vi "_ROSMasterConsole.vi"() -> ()   [LabVIEW 2012]
uses:
  <vilib>/Utility/miscctls.llb/LVRectTypeDef.ctl
  <userlib>/ROSforLV/ROS/Code/_ROSDefinition.vi
  <vilib>/Utility/cursorutil.llb/Set Cursor (Icon Pict).vi
panel:
  out "Servers Closed":bool[](array[boolean])
  in  "Stop":bool
  out "Error Log":string
  out "ROS Master":string="192.168.1.110:11311"
  out "selection":i32=-1
  out "2D Picture":picture
  out "Boundaries":cluster{i32, i32}[](array[cluster])=[{10, 22}, {30, 42}, {50, 62}]
  in  "expand?":bool
  out "Status":string
  out "Master?":bool
  out "Running?":bool
  out "current task":string
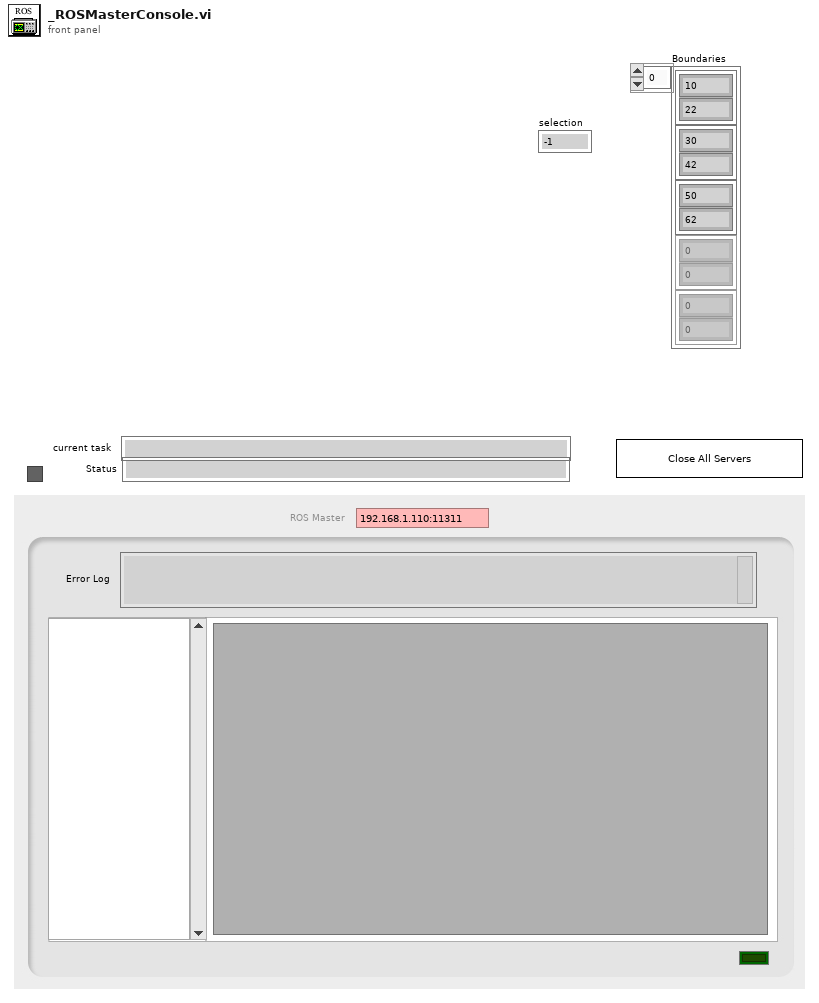
[diagram p1: front panel]
types:
  T1 = enum16{"Add Server", "Clear Server", "Clear All", "Get Info"}
  T2 = enum16{"Get Nodes", "Start Nodes", "Reset Nodes"}
  T3 = typedef "LVRectTypeDef.ctl" = cluster{"Left":i16, "Top":i16, "Right":i16, "Bottom":i16}
  T4 = typedef "_ROSControl.ctl" = cluster{"topic port":u16, "Node":string, "topic":string, "type":string, "node port":u32, "error ":errorcluster, "Direction":T5, "APIs":string[], "Update (ms)":u16, "write queue":u16}
  T5 = typedef "_ROSDirection.ctl" = enum16{"Node", "Publisher", "Subscriber", "Service Client"}
  T6 = typedef "ServoInfo.ctl" = cluster{"vi name":string, "VI Refnum":refnum<vi>, "queue":refnum<queue>, "ROS":T4, "notifier":refnum<notifier>}
  T7 = typedef "LVMouseTypeDef.ctl" = cluster{"Mouse Position":cluster{"X":i32, "Y":i32}, "Mouse Modifiers":cluster{"Button Down":bool, "Shift Mod":bool, "Menu Mod":bool, "Option Mod":bool}}
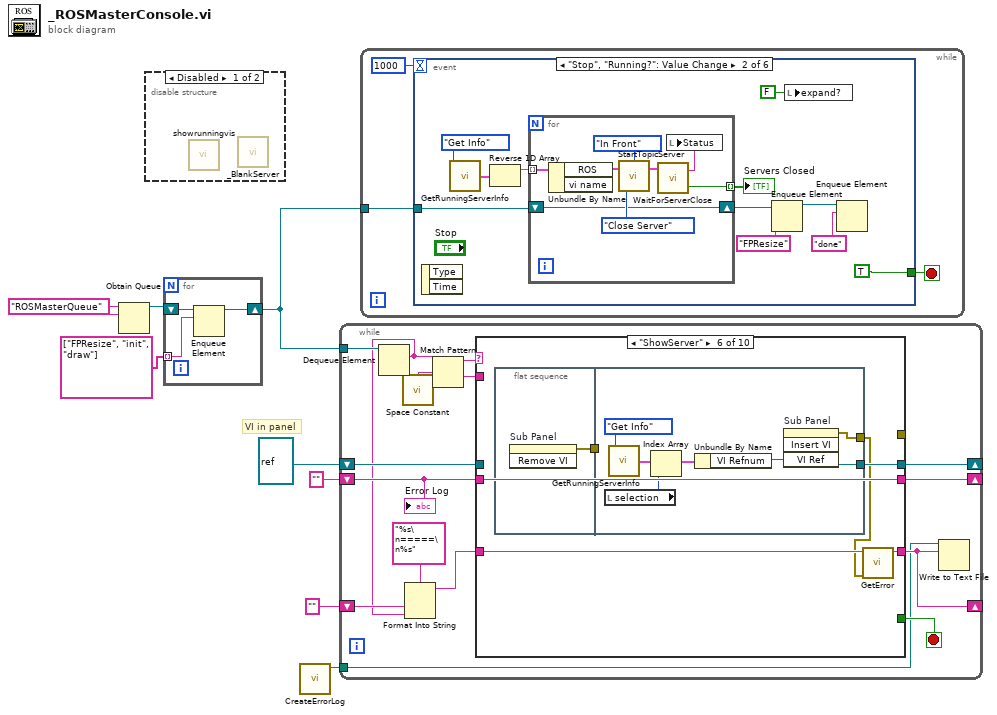
[diagram p0: block diagram]
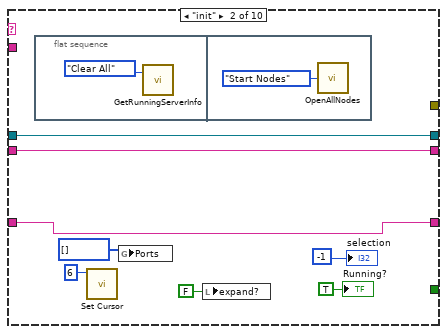
[diagram p4: hidden frame]
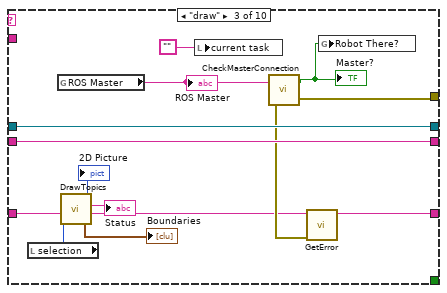
[diagram p5: hidden frame]
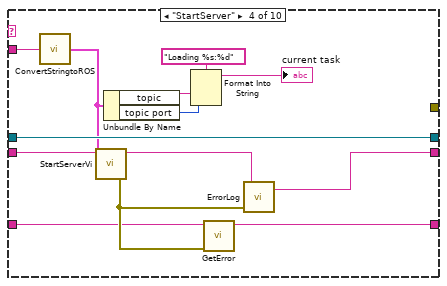
[diagram p6: hidden frame]
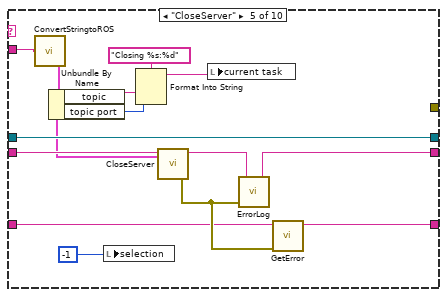
[diagram p7: hidden frame]
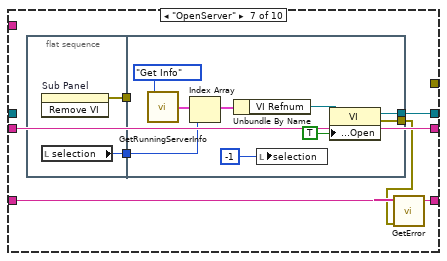
[diagram p8: hidden frame]
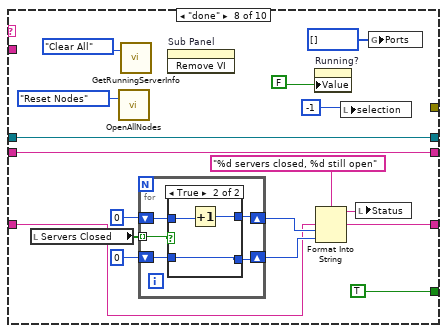
[diagram p9: hidden frame]
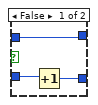
[diagram p10: hidden frame]
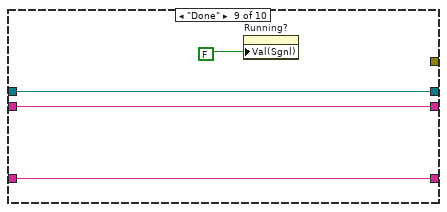
[diagram p11: hidden frame]
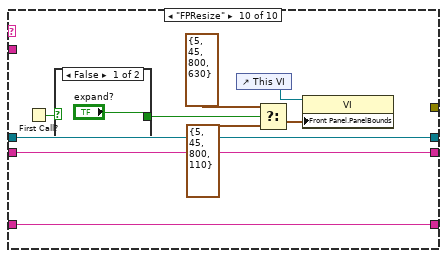
[diagram p12: hidden frame]
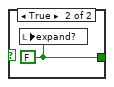
[diagram p13: hidden frame]
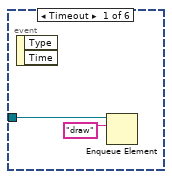
[diagram p14: hidden frame]
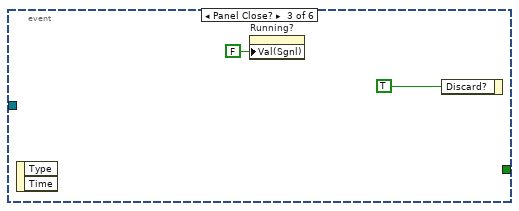
[diagram p15: hidden frame]
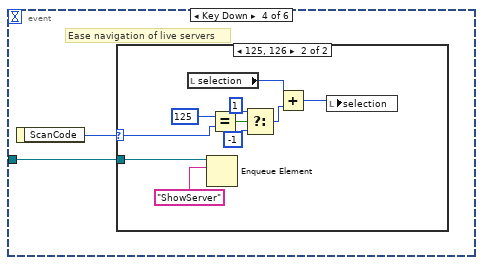
[diagram p16: hidden frame]
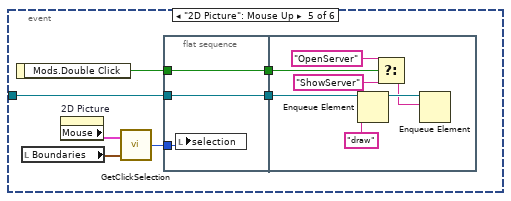
[diagram p18: hidden frame]
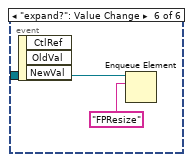
[diagram p19: hidden frame]
diagram:
  w8 = "ROSMasterQueue" ("name (unnamed)")
  # "VI in panel"
  n1 = Obtain Queue(name (unnamed)=w8, element data type=w8) -> (queue out=w5:refnum<queue>)  [unwired: 3 in, 2 out]
  n2 = disable-structure shown="Disabled" {
    frame Disabled {
      n3 = call <userlib>:"showrunningvis.vi"() -> ()  [unwired: 1 in]
      n4 = call <userlib>:"_BlankServer.vi"() -> ()  [unwired: 4 in]
    }
    frame Enabled {
    }
  }
  n5 = for {
    shift-right: [w11] -> w7
    shift-left: w5 -> [w10]
    tunnel: string[] ["FPResize", "init", "draw"] -> [w9] mode=indexing
    n6 = Enqueue Element(queue=w10, element=w9) -> (queue out=w11:refnum<queue>)  [unwired: 2 in, 2 out]
  }
  n7 = call <userlib>:"CreateErrorLog.vi"() -> ("path"=w1:path)  [unwired: 11 in]
  n8 = while {
    tunnel: w7 -> [w26]
    shift-right: [w20] -> _
    shift-left: refnum<vi> refnum ("VI Ref") -> [w21]
    shift-right: [w19] -> _
    shift-left: "" ("String out") -> [w18]
    shift-right: [w13] -> _
    shift-left: "" -> [w17]
    tunnel: w1 -> [w12]
    stop <- w25 stop-if-true
    n9 = Dequeue Element(queue=w26) -> (element=w15:string)  [unwired: 2 in, 3 out]
    n10 = call <vilib>:"Space Constant.vi"() -> ("String"=w23:string)
    n11 = Format Into String(format string="%s\n=====\n%s", w17, w15) -> (resulting string=w14:string)  [unwired: 2 in, 1 out]
    n12 = Match Pattern(string=w15, regular expression=w23) -> (before substring=w24:string, after substring=w22:string)  [unwired: 1 in, 2 out]
    n13 = case shown="\"ShowServer\"" w24 {
      tunnel: [_ _ _ _ _ _ _ TRUE _ _] -> w25
      tunnel: w22 -> [_ _ _ w60 w69 _ _ _ _ _]
      tunnel: w21 -> [w29 w37 w51 w63 w76 _ _ w122 w138 w147]
      tunnel: [w29 w37 w51 w63 w76 w81 w94 w122 w138 w147] -> w20
      tunnel: [_ _ w42 _ _ _ _ _ _ _] -> _
      tunnel: [w28 w31 w47 w55 w73 w80 w93 w117 w136 w140] -> w19
      tunnel: w18 -> [w28 w31 w47 w56 w74 w80 w93 w117 w136 w140]
      tunnel: w14 -> [w27 w30 w41 w53 w64 w78 w91 w108 w135 w139]
      tunnel: [w27 w30 w40 w52 w66 w79 w92 w108 w135 w139] -> w13
      frame Default {
      }
      frame "init" {
        n14 = flat-sequence {
          frame #0 {
            n15 = call <userlib>:"GetRunningServerInfo.vi"("Task"=T1."Clear All") -> ()  [unwired: 1 in, 3 out]
          }
          frame #1 {
            n16 = call <userlib>:"OpenAllNodes.vi"("Task"=T2."Start Nodes") -> ()  [unwired: 1 in, 1 out]
          }
        }
        n17 = call-poly <vilib>:"Set Cursor.vi"("icon"=u16 6) -> ()  [unwired: 9 in, 2 out]
        n18 = global write "_ROSDefinition.vi" "Ports"(u16[] [] ("Ports")) -> ()
        n19 = local write "expand?"(FALSE ("expand?")) -> ()
        "Running?" <- TRUE ("Running?")
        "selection" <- -1 ("selection")
      }
      frame "draw" {
        n20 = local read "selection"() -> (w50:i32)
        n21 = global read "_ROSDefinition.vi" "ROS Master"() -> (w45:string)
        "ROS Master" <- w45
        n22 = call <userlib>:"DrawTopics.vi"("Selection"=w50) -> ("new picture"=→"2D Picture":picture, "Status"=→"Status":string, "Boundaries"=→"Boundaries":cluster{i32, i32}[])  [unwired: 2 in, 1 out]
        n23 = local write "current task"("") -> ()
        n24 = call <userlib>:"CheckMasterConnection.vi"("Master IP"=w45) -> ("error out"=w42:errorcluster, "Master There?"=w43:bool)  [unwired: 1 in]
        "Master?" <- w43
        n25 = call <userlib>:"GetError.vi"("error in (no error)"=w42, "String in"=w41) -> ("String out"=w40:string)  [unwired: 9 in]
        n26 = global write "_ROSDefinition.vi" "Robot There?"(w43) -> ()
      }
      frame "StartServer" {
        n27 = call <userlib>:"ConvertStringtoROS.vi"("string in"=w60) -> ("ROS"=w57:T4)
        n28 = call <userlib>:"StartServerVi.vi"("ROS in"=w57) -> ("error out"=w54:errorcluster)  [unwired: 2 out]
        n29 = Unbundle By Name(w57) -> ("topic"=w59:string, "topic port"=w58:u16)
        n30 = Format Into String(format string="Loading %s:%d", w59, w58) -> (resulting string=→"current task":string)  [unwired: 2 in, 1 out]
        n31 = call <userlib>:"GetError.vi"("error in (no error)"=w54, "String in"=w53) -> ("String out"=w52:string)  [unwired: 9 in]
        n32 = call <userlib>:"ErrorLog.vi"("error in"=w54, "String in"=w56) -> ("String out"=w55:string)  [unwired: 1 in, 1 out]
      }
      frame "CloseServer" {
        n33 = call <userlib>:"ConvertStringtoROS.vi"("string in"=w69) -> ("ROS"=w67:T4)
        n34 = Unbundle By Name(w67) -> ("topic"=w71:string, "topic port"=w70:u16)
        n35 = local write "selection"(-1 ("Value (Signaling)")) -> ()
        n36 = Format Into String(format string="Closing %s:%d", w71, w70) -> (resulting string=w68:string)  [unwired: 2 in, 1 out]
        n37 = call <userlib>:"CloseServer.vi"("ROS"=w67) -> ("error out"=w65:errorcluster)  [unwired: 2 in]
        n38 = local write "current task"(w68) -> ()
        n39 = call <userlib>:"ErrorLog.vi"("error in"=w65, "String in"=w74) -> ("String out"=w73:string)  [unwired: 1 in, 1 out]
        n40 = call <userlib>:"GetError.vi"("error in (no error)"=w65, "String in"=w64) -> ("String out"=w66:string)  [unwired: 9 in]
      }
      frame "ShowServer" {
        n41 = flat-sequence {
          tunnel: [w83] -> w82
          tunnel: w82 -> [_]
          tunnel: [w89] -> w77
          tunnel: [w84] -> w81
          frame #0 {
            n42 = invoke on="Sub Panel" class="SubPanel" method="Remove VI"() -> (error out=w83:errorcluster)  [unwired: 3 in, 2 out]
          }
          frame #1 {
            n43 = local read "selection"() -> (w88:i32)
            n44 = call <userlib>:"GetRunningServerInfo.vi"("Task"=T1."Get Info") -> ("servers"=w86:T6[])  [unwired: 1 in, 2 out]
            n45 = Index Array(array=w86, index=w88) -> (element=w85:T6)
            n46 = Unbundle By Name(w85) -> ("VI Refnum"=w84:refnum<vi>)
            n47 = invoke on="Sub Panel" class="SubPanel" method="Insert VI"("VI Ref"=w84) -> (error out=w89:errorcluster)  [unwired: 3 in, 3 out]
          }
        }
        n48 = call <userlib>:"GetError.vi"("error in (no error)"=w77, "String in"=w78) -> ("String out"=w79:string)  [unwired: 9 in]
      }
      frame "OpenServer" {
        n49 = flat-sequence {
          tunnel: [w98] -> w96
          tunnel: [w97] -> w95
          tunnel: w96 -> [_]
          tunnel: w95 -> [w100]
          tunnel: [w105] -> w94
          tunnel: [w104] -> w90
          frame #0 {
            n50 = invoke on="Sub Panel" class="SubPanel" method="Remove VI"() -> (error out=w98:errorcluster)  [unwired: 3 in, 2 out]
            n51 = local read "selection"() -> (w97:i32)
          }
          frame #1 {
            n52 = call <userlib>:"GetRunningServerInfo.vi"("Task"=T1."Get Info") -> ("servers"=w102:T6[])  [unwired: 1 in, 2 out]
            n53 = Index Array(array=w102, index=w100) -> (element=w101:T6)
            n54 = Unbundle By Name(w101) -> ("VI Refnum"=w99:refnum<vi>)
            n55 = local write "selection"(-1 ("Live Servers")) -> ()
            n56 = property class="VI"(reference=w99, "Front Panel.Open"=TRUE ("Front Panel Window:Open")) -> (reference out=w105:refnum<vi>, error out=w104:errorcluster)  [unwired: 1 in]
          }
        }
        n57 = call <userlib>:"GetError.vi"("error in (no error)"=w90, "String in"=w91) -> ("String out"=w92:string)  [unwired: 9 in]
      }
      frame "done" {
        n58 = local read "Servers Closed"() -> (w116:bool[])
        n59 = call <userlib>:"OpenAllNodes.vi"("Task"=T2."Reset Nodes") -> ()  [unwired: 1 in, 1 out]
        n60 = call <userlib>:"GetRunningServerInfo.vi"("Task"=T1."Clear All") -> ()  [unwired: 1 in, 3 out]
        n61 = for {
          shift-right: [w126] -> w112
          shift-left: 0 -> [w127]
          shift-right: [w124] -> w111
          shift-left: 0 -> [w125]
          tunnel: w116 -> [w128] mode=indexing
          n62 = case shown="True" w128 {
            tunnel: w127 -> [w129 w134]
            tunnel: [w129 w133] -> w126
            tunnel: w125 -> [w131 w132]
            tunnel: [w130 w132] -> w124
            frame False {
              n63 = Increment(x=w131) -> (x+1=w130:i32)
            }
            frame True {
              n64 = Increment(x=w134) -> (x+1=w133:i32)
            }
          }
        }
        n65 = invoke on="Sub Panel" class="SubPanel" method="Remove VI"() -> ()  [unwired: 3 in, 3 out]
        n66 = property on="Running?" class="Bool (strict)"("Value"=FALSE) -> ()  [unwired: 2 in, 2 out]
        n67 = Format Into String(format string="%d servers closed, %d still open", w112, w111) -> (resulting string=w110:string)  [unwired: 2 in, 1 out]
        n68 = local write "selection"(-1 ("Live Servers")) -> ()
        n69 = local write "Status"(w110) -> ()
        n70 = global write "_ROSDefinition.vi" "Ports"(u16[] [] ("Ports")) -> ()
      }
      frame "Done" {
        n71 = property on="Running?" class="Bool (strict)"("Val(Sgnl)"=FALSE) -> ()  [unwired: 2 in, 2 out]
      }
      frame "FPResize" {
        n72 = First Call?() -> (First Call?: T/F=w142:bool)
        n73 = case shown="False" w142 {
          tunnel: ["expand?" w149] -> w141
          frame False {
          }
          frame True {
            w149 = FALSE ("expand?")
            n74 = local write "expand?"(w149) -> ()
          }
        }
        n75 = control-ref of="This VI"() -> (w146:refnum<vi>)
        n76 = Select(t=T3 {"Left"=5, "Top"=45, "Right"=800, "Bottom"=630} ("Front Panel Window:Panel Bounds"), s=w141, f=T3 {"Left"=5, "Top"=45, "Right"=800, "Bottom"=110} ("Front Panel Window:Panel Bounds")) -> (s? t:f=w144:T3)
        n77 = property class="VI"(reference=w146, "Front Panel.PanelBounds"=w144) -> ()  [unwired: 1 in, 2 out]
      }
    }
    n78 = Write to Text File(file (use dialog)=w12, text=w13) -> ()  [unwired: 2 in, 3 out]
    "Error Log" <- w18
  }
  n79 = while {
    tunnel: w7 -> [w152]
    stop <- w151 stop-if-true
    n80 = event shown="[1] \"Stop\", \"Running?\": Value Change" {
      selector: _ -> [_ _ _ _ _ _]
      dyn-events: _ -> [_ _ _ _ _ _]
      timeout: 1000 -> [_ _ _ _ _ _]
      tunnel: w152 -> [w154 w164 _ w177 w194 w205]
      tunnel: [_ TRUE ("Stop") _ _ _ _] -> w151
      event Timeout {
        n81 = event-data() -> ()  [unwired: 1 in, 2 out]
        n82 = Enqueue Element(queue=w154, element="draw") -> ()  [unwired: 2 in, 3 out]
      }
      event "Stop", "Running?": Value Change {
        n83 = event-data() -> ()  [unwired: 1 in, 2 out]
        n84 = call <userlib>:"GetRunningServerInfo.vi"("Task"=T1."Get Info") -> ("servers"=w156:T6[])  [unwired: 1 in, 2 out]
        n85 = Reverse 1D Array(array=w156) -> (reversed array=w157:T6[])
        n86 = for {
          shift-right: [w169] -> w161
          shift-left: w164 -> [w169]
          tunnel: w157 -> [w173] mode=indexing
          tunnel: [w166] -> w155 mode=indexing
          n87 = Unbundle By Name(w173) -> ("ROS"=w170:T4)  [unwired: 1 out]
          n88 = call <userlib>:"StartTopicServer.vi"("Server Direction"=enum16{"Start Server", "Close Server"}."Close Server", "ROS in"=w170, "Priority"=enum16{"In Front", "In Back"}."In Front") -> ("ROS out"=w168:T4)  [unwired: 1 in]
          n89 = call <userlib>:"WaitForServerClose.vi"("ROS in"=w168) -> ("Closed"=w166:bool, "resulting string"=w167:string)  [unwired: 1 in]
          n90 = local write "Status"(w167) -> ()
        }
        "Servers Closed" <- w155
        n91 = Enqueue Element(queue=w161, element="FPResize") -> (queue out=w160:refnum<queue>)  [unwired: 2 in, 2 out]
        n92 = local write "expand?"(FALSE ("expand?")) -> ()
        n93 = Enqueue Element(queue=w160, element="done") -> ()  [unwired: 2 in, 3 out]
      }
      event Panel Close? {
        n94 = event-data() -> ()  [unwired: 1 in, 2 out]
        n95 = property on="Running?" class="Bool (strict)"("Val(Sgnl)"=FALSE ("Value (Signaling)")) -> ()  [unwired: 2 in, 2 out]
        n96 = event-data("Discard?"=TRUE ("Stop")) -> ()  [unwired: 1 in, 1 out]
      }
      event Key Down {
        # "Ease navigation of live servers"
        n97 = event-data() -> ("ScanCode"=w176:i16)  [unwired: 1 in]
        n98 = case shown="125, 126" w176 {
          selector: w176 -> [_ w185]
          tunnel: w177 -> [_ w187]
          frame Default {
          }
          frame 125, 126 {
            n99 = local read "selection"() -> (w178:i32)
            n100 = Enqueue Element(queue=w187, element="ShowServer") -> ()  [unwired: 2 in, 3 out]
            n101 = Equal?(x=i16 125, y=w185) -> (x = y?=w183:bool)
            n102 = Select(t=i16 1 ("x"), s=w183, f=i16 -1 ("x")) -> (s? t:f=w182:i16)
            n103 = Add(x=w178, y=w182) -> (x+y=w179:i32)
            n104 = local write "selection"(w179) -> ()
          }
        }
      }
      event "2D Picture": Mouse Up {
        n105 = event-data() -> ("Mods.Double Click"=w191:bool)  [unwired: 1 in]
        n106 = local read "Boundaries"() -> (w192:cluster{i32, i32}[])
        n107 = property on="2D Picture" class="Pict"() -> ("Mouse"=w193:T7)  [unwired: 2 in, 2 out]
        n108 = call <userlib>:"GetClickSelection.vi"("Boundaries"=w192, "Mouse"=w193) -> ("selection"=w188:i32)
        n109 = flat-sequence {
          tunnel: w191 -> [w196]
          tunnel: w194 -> [w197]
          tunnel: [w197] -> w190
          tunnel: [w196] -> w189
          tunnel: w188 -> [w195]
          tunnel: w190 -> [w203]
          tunnel: w189 -> [w202]
          frame #0 {
            n110 = local write "selection"(w195) -> ()
          }
          frame #1 {
            n111 = Enqueue Element(queue=w203, element="draw" ("name (unnamed)")) -> (queue out=w199:refnum<queue>)  [unwired: 2 in, 2 out]
            n112 = Select(t="OpenServer" ("element"), s=w202, f="ShowServer" ("element")) -> (s? t:f=w198:string)
            n113 = Enqueue Element(queue=w199, element=w198) -> ()  [unwired: 2 in, 3 out]
          }
        }
      }
      event "expand?": Value Change {
        n114 = event-data() -> ()  [unwired: 1 in, 3 out]
        n115 = Enqueue Element(queue=w205, element="FPResize") -> ()  [unwired: 2 in, 3 out]
      }
    }
  }
